vi "Part 2.vi"(11 "Input":string) -> (3 "Output":i64)   [LabVIEW 2021]
uses:
  49c6387d-53bd-456a-b0f5-19eb8014877a.vi
  <userlib>/_OpenG.lib/string/string.llb/Convert EOLs (String)__ogtk.vi
  <vilib>/Comparison/Equal/Equal Functor/Equal Functor.lvclass
panel:
  out "Map":string[][](array[string])
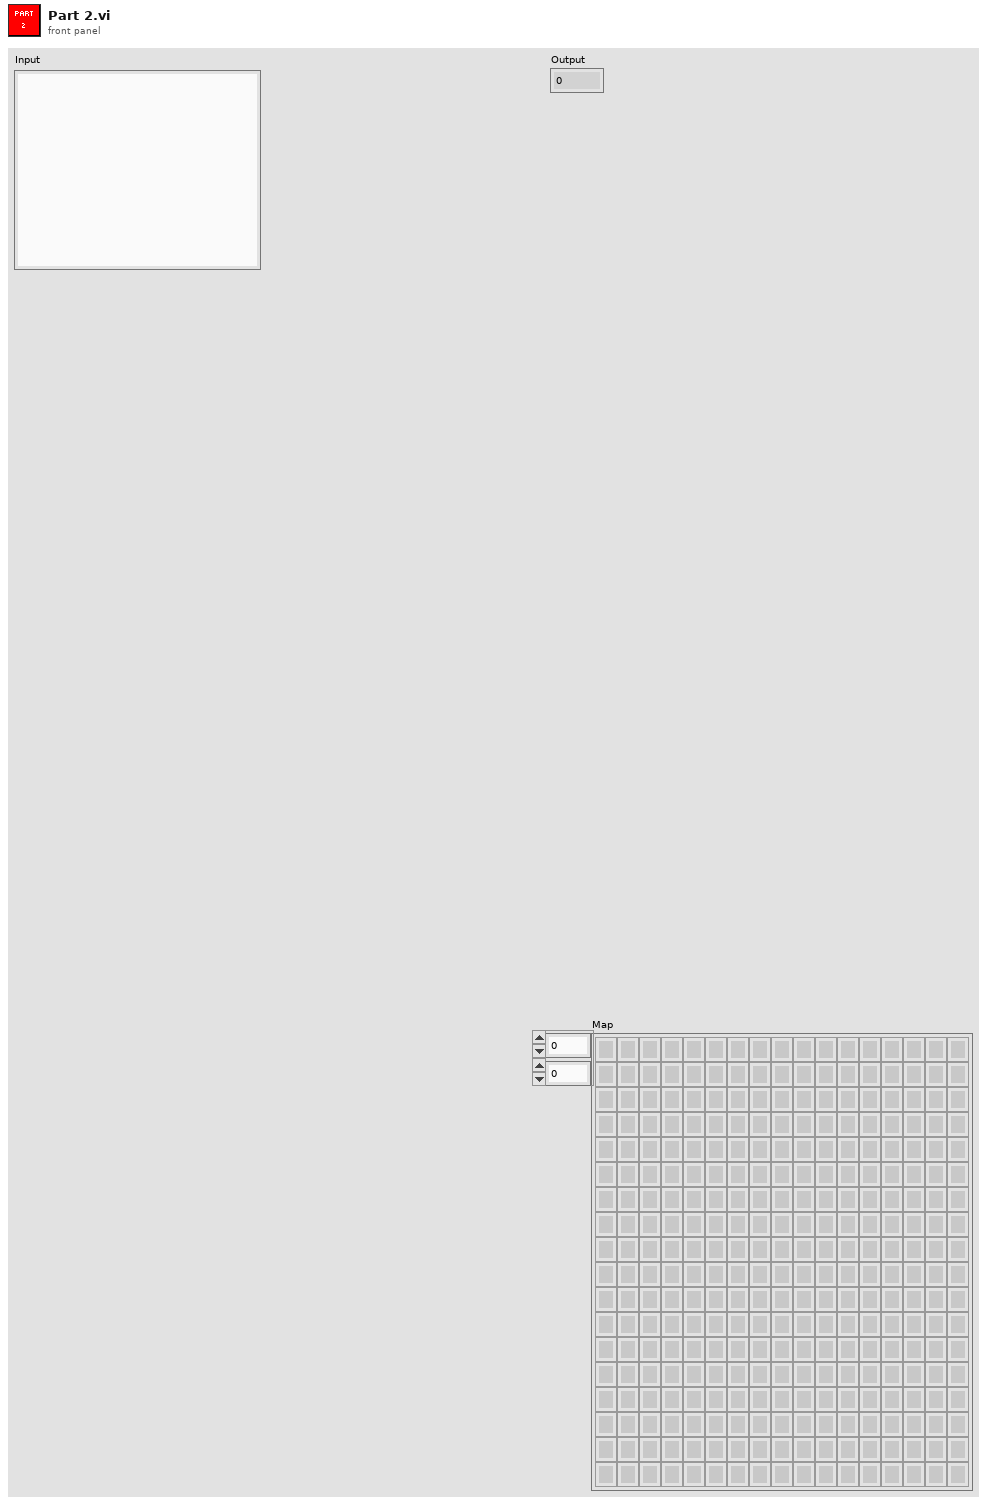
[diagram p1: front panel]
types:
  T1 = set{cluster{"Row":i32, "Col":i32, "Direction":i32}}
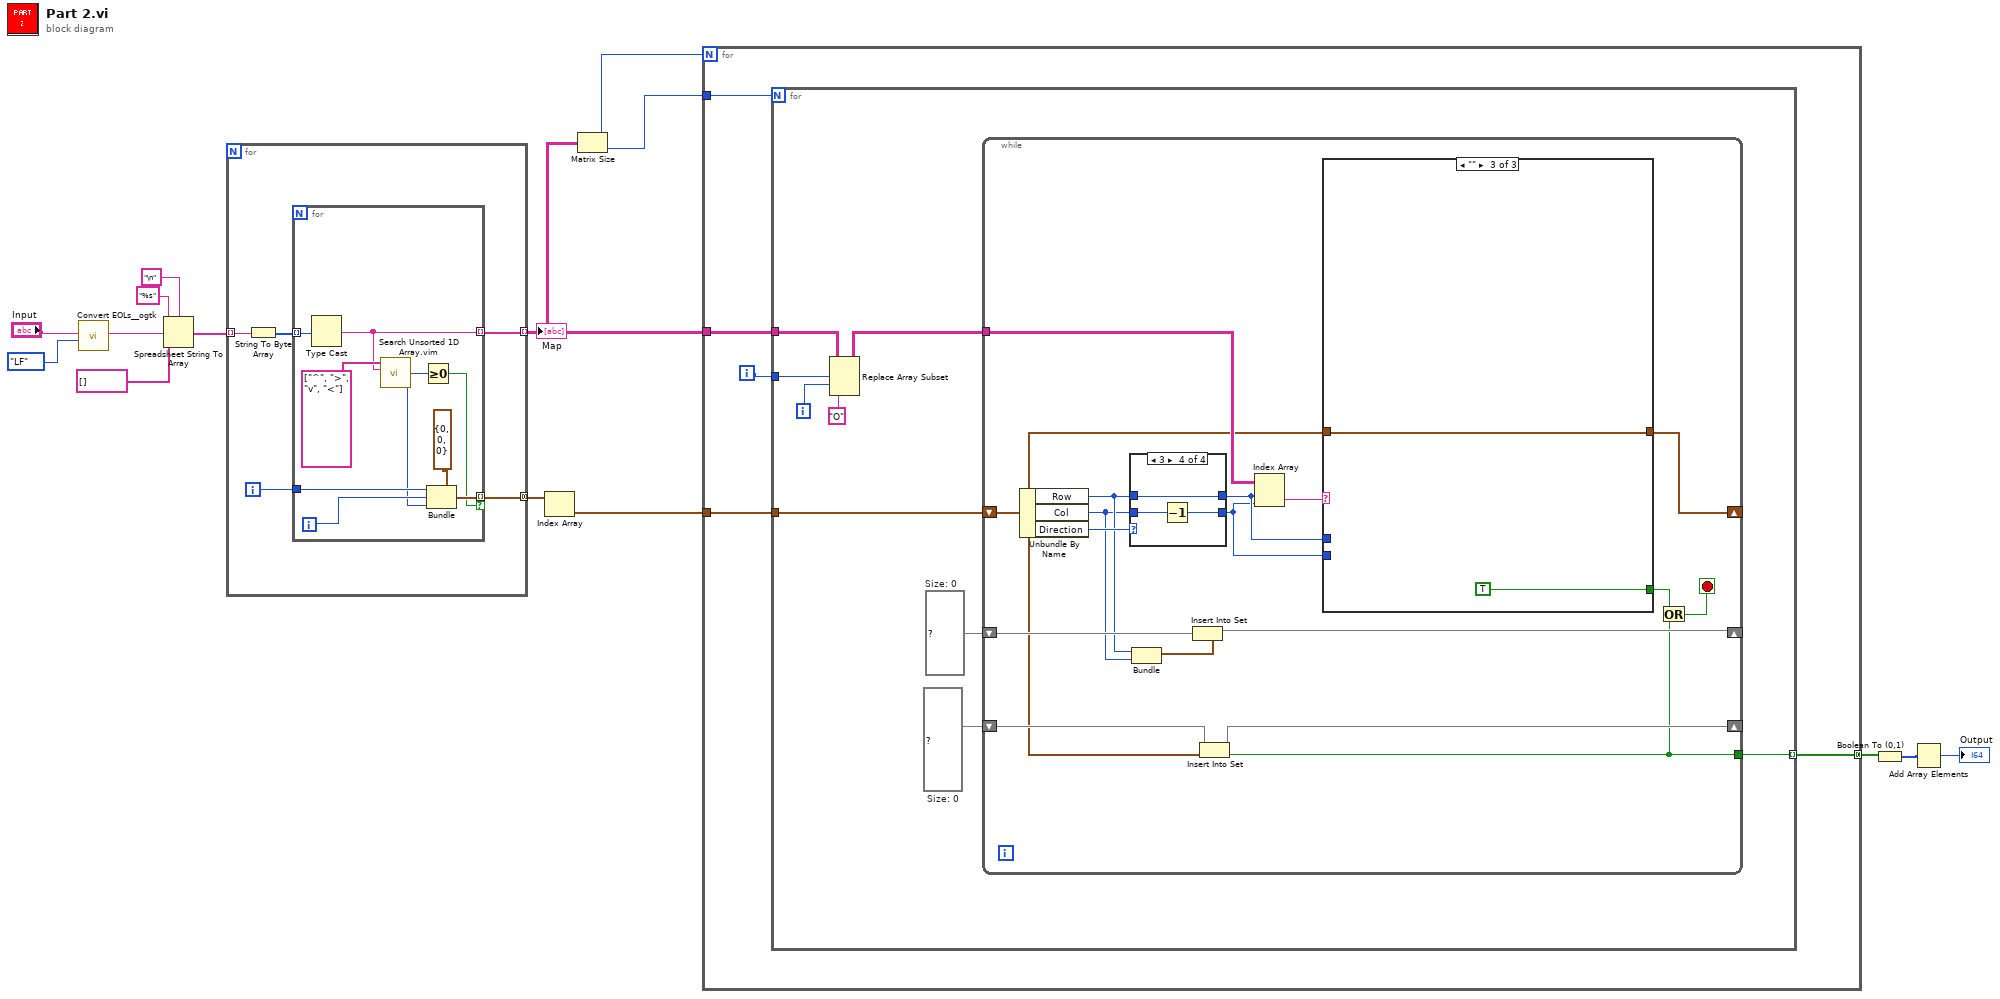
[diagram p0: block diagram]
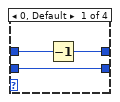
[diagram p2: hidden frame]
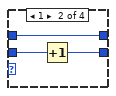
[diagram p3: hidden frame]
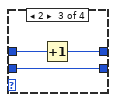
[diagram p4: hidden frame]
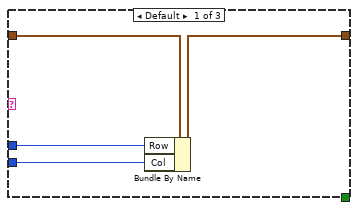
[diagram p5: hidden frame]
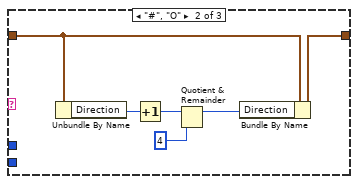
[diagram p6: hidden frame]
diagram:
  n1 = call-poly <userlib>:"Convert EOLs__ogtk.vi"("Convert to:"=enum16{"CR", "LF", "CRLF"}."LF", "String in"="Input") -> ("String out"=w12:string)  [unwired: 9 in]
  n2 = Spreadsheet String To Array(delimiter (Tab)="\n", format string="%s", spreadsheet string=w12, array type (2D Dbl)=string[] []) -> (array=w10:string[])
  n3 = for {
    tunnel: w10 -> [w20] mode=indexing
    tunnel: [w18] -> w6 mode=indexing
    tunnel: [w16] -> w9 mode=concatenating
    i -> [w17]
    n4 = String To Byte Array(string=w20) -> (unsigned byte array=w19:u8[])
    n5 = for {
      tunnel: w19 -> [w29] mode=indexing
      tunnel: [w22] -> w18 mode=indexing
      tunnel: w17 -> [w28]
      tunnel: [w24] -> w16 mode=indexing if=w23
      i -> [w27]
      n6 = Type Cast(x=w29) -> (*(type *) &x=w22:string)  [unwired: 1 in]
      n7 = call "Search Unsorted 1D Array.vim"("element"=w22, "unsorted 1D array"=string[] ["^", ">", "v", "<"]) -> ("index of element"=w25:i32)  [unwired: 9 in]
      n8 = Greater Or Equal To 0?(x=w25) -> (x >= 0?=w23:bool)
      n9 = Bundle(cluster=cluster{"Row":i32, "Col":i32, "Direction":i32} {"Row"=0, "Col"=0, "Direction"=0} ("Position"), "Row"=w28, "Col"=w27, "Direction"=w25) -> (w24:cluster{"Row":i32, "Col":i32, "Direction":i32})
    }
  }
  "Map" <- w6
  n10 = Index Array(array=w9) -> (element=w8:cluster{"Row":i32, "Col":i32, "Direction":i32})  [unwired: 1 in]
  n11 = Matrix Size(0:w6) -> (1:w5:i32, 2:w4:i32)
  n12 = for {
    N: w5 -> [_]
    tunnel: w8 -> [w34]
    tunnel: w6 -> [w33]
    tunnel: w4 -> [w32]
    tunnel: [w30] -> w3 mode=concatenating
    i -> [w31]
    n13 = for {
      N: w32 -> [_]
      tunnel: w34 -> [w43]
      tunnel: w33 -> [w39]
      tunnel: w31 -> [w38]
      tunnel: [w35] -> w30 mode=indexing
      i -> [w37]
      w41 = T1 {}  # Size: 0
      w42 = set{cluster{"Row":i32, "Col":i32}} {}  # Size: 0
      n14 = Replace Array Subset(array=w39, new element="O", index (row)=w38, index (col)=w37) -> (w40:string[][])
      n15 = while {
        shift-right: [w52] -> _
        shift-left: w43 -> [w48]
        shift-right: [w53] -> _
        shift-left: w42 -> [w57]
        tunnel: w40 -> [w59]
        shift-right: [w47] -> _
        shift-left: w41 -> [w49]
        tunnel: [w44] -> w35
        stop <- w45 stop-if-true
        n16 = Unbundle By Name(w48) -> ("Row"=w56:i32, "Col"=w55:i32, "Direction"=w60:i32)
        n17 = case shown="3" w60 {
          tunnel: w55 -> [w63 w66 w68 w72]
          tunnel: w56 -> [w62 w65 w69 w71]
          tunnel: [w63 w64 w68 w70] -> w50
          tunnel: [w61 w65 w67 w71] -> w51
          frame 0, Default {
            n18 = Decrement(x=w62) -> (x-1=w61:i32)
          }
          frame 1 {
            n19 = Increment(x=w66) -> (x+1=w64:i32)
          }
          frame 2 {
            n20 = Increment(x=w69) -> (x+1=w67:i32)
          }
          frame 3 {
            n21 = Decrement(x=w72) -> (x-1=w70:i32)
          }
        }
        n22 = Bundle("Row"=w56, "Col"=w55) -> (w54:cluster{"Row":i32, "Col":i32})  [unwired: 1 in]
        n23 = Insert Into Set(10:w54, 11:w57) -> (3:w53:set{cluster{"Row":i32, "Col":i32}})  [unwired: 1 out]
        n24 = Insert Into Set(10:w48, 11:w49) -> (2:w44:bool, 3:w47:T1)
        n25 = Index Array(array=w59, index (row)=w51, index (col)=w50) -> (element=w58:string)
        n26 = case shown="\"\"" w58 {
          tunnel: [_ _ TRUE] -> w46
          tunnel: w48 -> [w76 w81 w83]
          tunnel: [w75 w82 w83] -> w52
          tunnel: w51 -> [w74 _ _]
          tunnel: w50 -> [w73 _ _]
          frame Default {
            n27 = Bundle By Name(cluster=w76, "Row"=w74, "Col"=w73) -> (w75:cluster{"Row":i32, "Col":i32, "Direction":i32})
          }
          frame "#", "O" {
            n28 = Unbundle By Name(w81) -> ("Direction"=w80:i32)
            n29 = Increment(x=w80) -> (x+1=w79:i32)
            n30 = Quotient & Remainder(x=w79, y=4) -> (x-y*floor(x/y)=w78:i32)  [unwired: 1 out]
            n31 = Bundle By Name(cluster=w81, "Direction"=w78) -> (w82:cluster{"Row":i32, "Col":i32, "Direction":i32})
          }
          frame "" {
          }
        }
        n32 = Or(x=w46, y=w44) -> (x .or. y?=w45:bool)
      }
    }
  }
  n33 = Boolean To (0,1)(Boolean=w3) -> (0, 1=w2:i16[])
  n34 = Add Array Elements(numeric array=w2) -> (sum=→"Output":i16)
